vi "OpenBase.vi"(5 "LogEnabled":bool, 7 "LogPath":path, 8 "error in (no error)":errorcluster, 9 "Instance":string, 10 "BaudRate":u32=125000, 11 "National Instruments USB-8473 Adapter Class in":refnum<class "National Instruments USB-8473 Adapter Class.lvclass">) -> (0 "error out":errorcluster, 3 "National Instruments USB-8473 Adapter Class out":refnum<class "National Instruments USB-8473 Adapter Class.lvclass">)   [LabVIEW 2011, in "National Instruments USB-8473 Adapter Class.lvclass"]
uses:
  National Instruments USB-8473 Adapter Class.lvclass
  <vilib>/nican/nican.llb/ncNetAttr.ctl
  National Instruments USB-8473 Adapter Class.lvclass/National Instruments USB-8473 Adapter Class.ctl
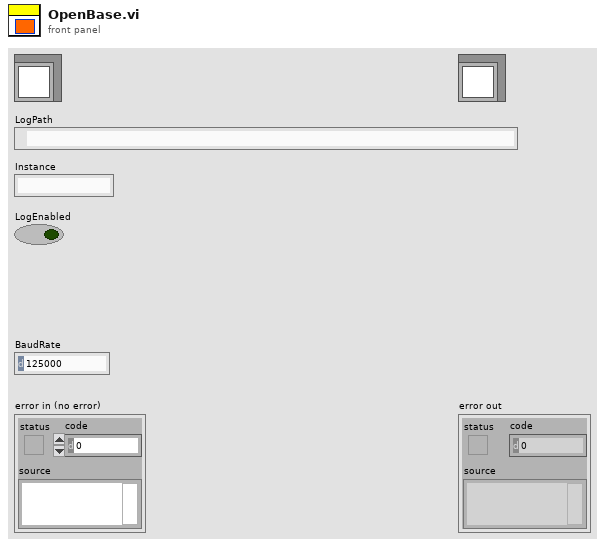
[diagram p1: front panel]
types:
  T1 = typedef "ncNetAttr.ctl" = cluster{"Start On Open":enum32{"FALSE", "TRUE"}, "Baud Rate":u32, "Read Queue Length":u32, "Write Queue Length":u32, "Standard Comparator":u32, "Standard Mask":u32, "Extended Comparator":u32, "Extended Mask":u32}
  T2 = typedef "xobjhandle.ctl" = u32
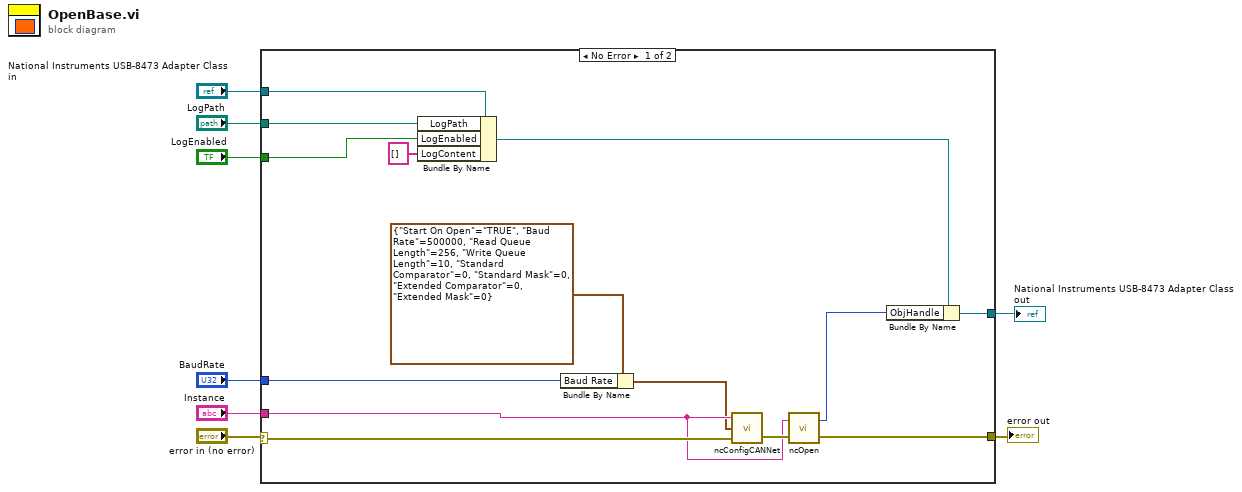
[diagram p0: block diagram]
diagram:
  n1 = case shown="No Error" "error in (no error)" {
    selector: "error in (no error)" -> [w21 w24]
    tunnel: "National Instruments USB-8473 Adapter Class in" -> [w22 w23]
    tunnel: [w18 w24] -> w6
    tunnel: "LogPath" -> [w20 _]
    tunnel: "LogEnabled" -> [w10 _]
    tunnel: "Instance" -> [w17 _]
    tunnel: "BaudRate" -> [w14 _]
    tunnel: [w12 w23] -> w1
    frame No Error {
      n2 = Bundle By Name(cluster=w22, "LogPath"=w20, "LogEnabled"=w10, "LogContent"=string[] []) -> (w13:refnum<class "National Instruments USB-8473 Adapter Class.lvclass">)
      n3 = Bundle By Name(cluster=T1 {"Start On Open"=enum."TRUE", "Baud Rate"=500000, "Read Queue Length"=256, "Write Queue Length"=10, "Standard Comparator"=0, "Standard Mask"=0, "Extended Comparator"=0, "Extended Mask"=0} ("CAN Network Interface Config"), "Baud Rate"=w14) -> (w15:T1)
      n4 = call <vilib>:"ncConfigCANNet.vi"("Error in"=w21, "CAN Network Interface Config"=w15, "ObjName"=w17) -> ("Error out"=w19:errorcluster)  [unwired: 2 in]
      n5 = call <vilib>:"ncOpen.vi"("Error in"=w19, "ObjName"=w17) -> ("Error out"=w18:errorcluster, "ObjHandle out"=w11:T2)
      n6 = Bundle By Name(cluster=w13, "ObjHandle"=w11) -> (w12:refnum<class "National Instruments USB-8473 Adapter Class.lvclass">)
    }
    frame Error {
    }
  }
  "National Instruments USB-8473 Adapter Class out" <- w1
  "error out" <- w6
